vi "nanomsg_sendmsg.vi"(3 "error in":errorcluster, 4 "no block? (F)":bool, 5 "parts":string[](array[string]), 6 "socket in":refnum<class "nanomsg_socket.lvclass">) -> (0 "error out":errorcluster, 2 "socket out":refnum<class "nanomsg_socket.lvclass">)   [LabVIEW 2014, in "nanomsg.lvlib" / "nanomsg_socket.lvclass"]
doc: "Sends a multi-component message corresponding to the elements of <b>parts</b> through the socket."
uses:
  nanomsg_socket.lvclass
  nanomsg_socket.lvclass/nanomsg_socket.ctl
  <vilib>/Utility/error.llb/Error Cluster From Error Code.vi
  nanomsg.lvlib
panel:
  # "NN"
  # "labview"
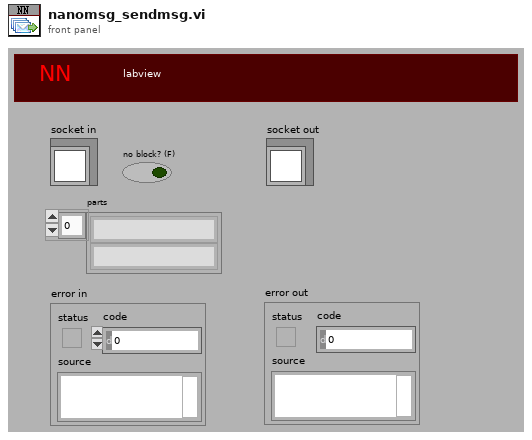
[diagram p1: front panel]
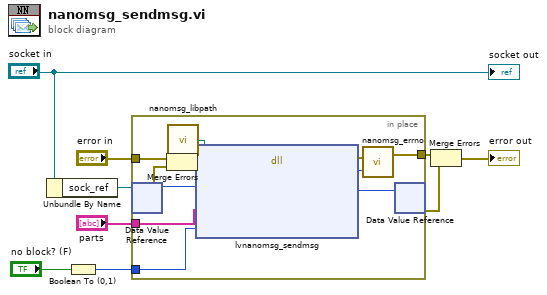
[diagram p0: block diagram]
diagram:
  n1 = Unbundle By Name("socket in") -> ("sock_ref"=w5:refnum<data-value>)
  n2 = Boolean To (0,1)(Boolean="no block? (F)") -> (0, 1=w1:i16)
  n3 = in-place {
    in-place-border: "parts" -> [w18]
    in-place-border: "error in" -> [w17]
    in-place-border: [w16] -> w7
    in-place-border: w1 -> [w10]
    n4 = in-place-dvr #1(w5) -> (w15:u64, w11:errorcluster)
    n5 = Merge Errors(w17, w11) -> (w12:errorcluster)
    n6 = call "nanomsg_libpath.vi"() -> ("path"=w13:path)
    n7 = dll-call lib="?" fn="lvnanomsg_sendmsg" ("zmq_labview.dll:lvzmq_socket")(path in=w13, error in=w12, "sock_obj"=w15, "data"=w18, "flags"=w10) -> (error out=w20:errorcluster, "return type"=w19:i32, "sock_obj"=w14:u64)  [unwired: 3 in, 1 out]
    n8 = call "nanomsg_errno.vi"("retval"=w19, "error in"=w20) -> ("error out"=w16:errorcluster)  [unwired: 1 out]
    n9 = in-place-dvr #1(w14) -> (w3:errorcluster)  [unwired: 1 out]
  }
  n10 = Merge Errors(w7, w3) -> (→"error out":errorcluster)
  "socket out" <- "socket in"
